vi "Start Async.vi"(8 "error in (no error)":errorcluster, 11 "gRPC Server in":refnum<class "NiDAQmx.lvclass">) -> (0 "error out":errorcluster, 3 "gRPC Server out":refnum<class "NiDAQmx.lvclass">)   [LabVIEW 2021, in "NI DAQmx_server.lvlib" / "NiDAQmx.lvclass"]
uses:
  NiDAQmx.lvclass
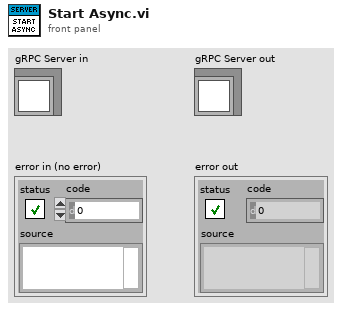
[diagram p1: front panel]
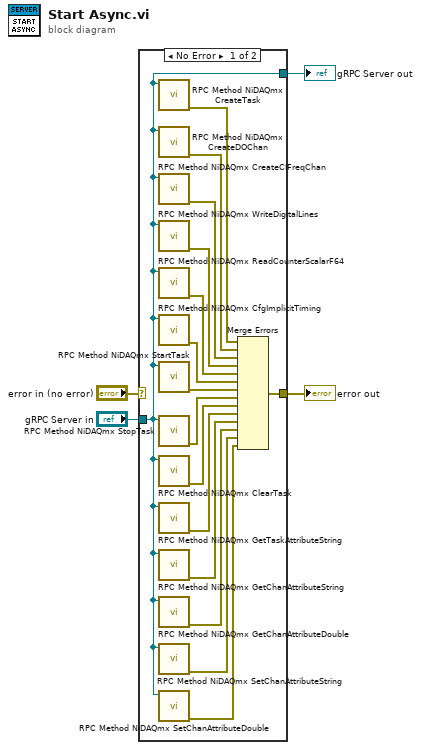
[diagram p0: block diagram]
diagram:
  n1 = case shown="No Error" "error in (no error)" {
    selector: "error in (no error)" -> [_ w22]
    tunnel: [w20 w22] -> w3
    tunnel: [w19 w21] -> w1
    tunnel: "gRPC Server in" -> [w19 w21]
    frame No Error {
      n2 = call "RPC Method NiDAQmx CreateTask.vi"("OOP Server in"=w19) -> ("error out"=w18:errorcluster)  [unwired: 9 in, 1 out]
      n3 = call "RPC Method NiDAQmx CreateDOChan.vi"("OOP Server in"=w19) -> ("error out"=w17:errorcluster)  [unwired: 9 in, 1 out]
      n4 = call "RPC Method NiDAQmx CreateCIFreqChan.vi"("OOP Server in"=w19) -> ("error out"=w16:errorcluster)  [unwired: 9 in, 1 out]
      n5 = call "RPC Method NiDAQmx WriteDigitalLines.vi"("OOP Server in"=w19) -> ("error out"=w15:errorcluster)  [unwired: 9 in, 1 out]
      n6 = call "RPC Method NiDAQmx ReadCounterScalarF64.vi"("OOP Server in"=w19) -> ("error out"=w14:errorcluster)  [unwired: 9 in, 1 out]
      n7 = call "RPC Method NiDAQmx CfgImplicitTiming.vi"("OOP Server in"=w19) -> ("error out"=w13:errorcluster)  [unwired: 9 in, 1 out]
      n8 = call "RPC Method NiDAQmx StartTask.vi"("OOP Server in"=w19) -> ("error out"=w12:errorcluster)  [unwired: 9 in, 1 out]
      n9 = call "RPC Method NiDAQmx StopTask.vi"("OOP Server in"=w19) -> ("error out"=w11:errorcluster)  [unwired: 9 in, 1 out]
      n10 = call "RPC Method NiDAQmx ClearTask.vi"("OOP Server in"=w19) -> ("error out"=w10:errorcluster)  [unwired: 9 in, 1 out]
      n11 = call "RPC Method NiDAQmx GetTaskAttributeString.vi"("OOP Server in"=w19) -> ("error out"=w9:errorcluster)  [unwired: 9 in, 1 out]
      n12 = call "RPC Method NiDAQmx GetChanAttributeString.vi"("OOP Server in"=w19) -> ("error out"=w8:errorcluster)  [unwired: 9 in, 1 out]
      n13 = call "RPC Method NiDAQmx GetChanAttributeDouble.vi"("OOP Server in"=w19) -> ("error out"=w7:errorcluster)  [unwired: 9 in, 1 out]
      n14 = call "RPC Method NiDAQmx SetChanAttributeString.vi"("OOP Server in"=w19) -> ("error out"=w6:errorcluster)  [unwired: 9 in, 1 out]
      n15 = call "RPC Method NiDAQmx SetChanAttributeDouble.vi"("OOP Server in"=w19) -> ("error out"=w5:errorcluster)  [unwired: 9 in, 1 out]
      n16 = Merge Errors(w18, w17, w16, w15, w14, w13, w12, w11, w10, w9, w8, w7, w6, w5) -> (w20:errorcluster)
    }
    frame Error {
    }
  }
  "error out" <- w3
  "gRPC Server out" <- w1
